vi "Decimate Waveform Absolute.vi"(6 "Width":u32, 8 "error in (no error)":errorcluster, 9 "Xmin":dbl, 10 "Xmax":dbl, 11 "Data to Decimate":waveform(dbl)[](array[waveform])) -> (0 "error out":errorcluster, 3 "Decimated Data":waveform(dbl)[](array[waveform]))   [LabVIEW 2022 SP3, in "Decimation.lvlib"]
doc: "Decimate waveform array to optimize the density of points per pixel to 2 : Min & Max per pixel."
uses:
  Decimation.lvlib
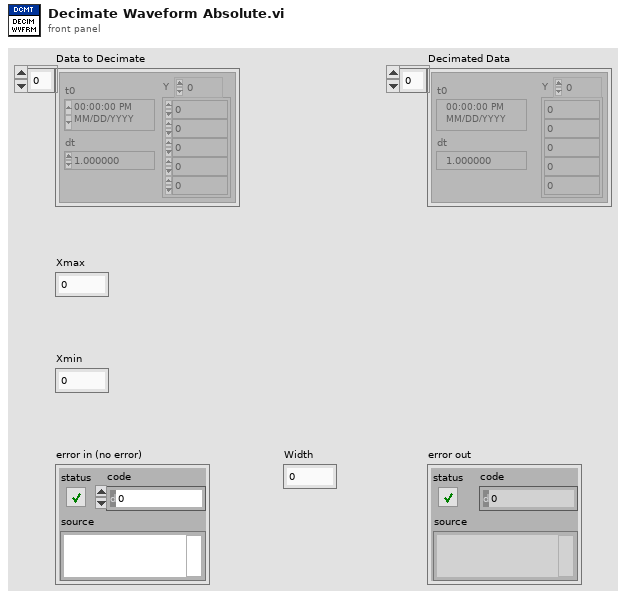
[diagram p1: front panel]
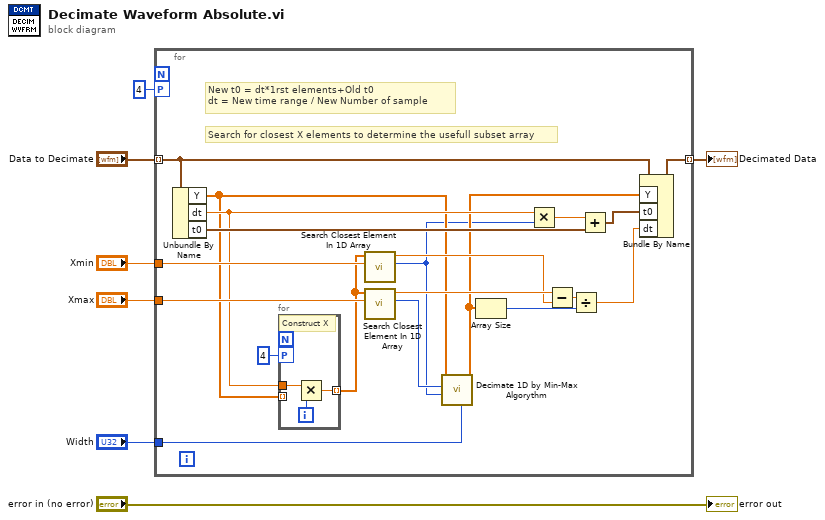
[diagram p0: block diagram]
diagram:
  n1 = for {
    tunnel: "Data to Decimate" -> [w21] mode=indexing
    tunnel: "Xmin" -> [w27]
    tunnel: "Xmax" -> [w26]
    tunnel: "Width" -> [w13]
    tunnel: [w25] -> w4 mode=indexing
    workers-P: 4 -> [_]
    # "New t0 = dt*1rst elements+Old t0\ndt = New time range / New Number of sample"
    # "Search for closest X elements to determine the usefull subset array"
    n2 = Unbundle By Name(w21) -> ("Y"=w12:dbl[], "dt"=w19:dbl, "t0"=w23:timestamp)
    n3 = for {
      tunnel: w19 -> [w30]
      tunnel: [w28] -> w20 mode=indexing
      tunnel: w12 -> [_] mode=indexing
      workers-P: 4 -> [_]
      i -> [w29]
      # "Construct X"
      n4 = Multiply(x=w30, y=w29) -> (x*y=w28:dbl)
    }
    n5 = call "Search Closest Element In 1D Array.vi"("Desired element"=w27, "1D Array"=w20) -> ("Closest Index"=w9:i32, "Closest Element"=w17:dbl)  [unwired: 8 in]
    n6 = call "Search Closest Element In 1D Array.vi"("Desired element"=w26, "1D Array"=w20) -> ("Closest Index"=w10:i32, "Closest Element"=w18:dbl)  [unwired: 8 in]
    n7 = call "Decimate 1D by Min-Max Algorythm.vi"("Width"=w13, "Min Index"=w9, "Max Index"=w10, "Data To Decimate"=w12) -> ("Decimated Data"=w11:dbl[])  [unwired: 6 in, 1 out]
    n8 = Array Size(array=w11) -> (size(s)=w14:i32)
    n9 = Multiply(x=w19, y=w9) -> (x*y=w24:dbl)
    n10 = Subtract(x=w18, y=w17) -> (x-y=w16:dbl)
    n11 = Divide(x=w16, y=w14) -> (x/y=w15:dbl)
    n12 = Add(x=w24, y=w23) -> (x+y=w22:timestamp)
    n13 = Bundle By Name(cluster=w21, "Y"=w11, "t0"=w22, "dt"=w15) -> (w25:waveform(dbl))
  }
  "Decimated Data" <- w4
  "error out" <- "error in (no error)"
